vi "MGI RWA Unprocess Array Elements.vi"(0 "Queue In":refnum<queue>, 1 "Value":string, 2 "Read/Write Options":T2={"TS Fmt"="", "Int Fmt"="", "Delimiter"=","}, 3 "Format String (%#_13g)":string="%#_13g", 5 "Array Variant":variant, 7 "Name In":string, 9 "Str to INI in":variant, 11 "Error In":errorcluster, 12 "Use Specified?":bool, 13 "State In":T1={"StrToSpecifiedText"=variant, "Specified Data"=variant, "Float Fmt"="%#_13g", "Major Vers"=0, "Options"={"TS Fmt"="", "Int Fmt"="", "Delimiter"=","}}) -> (4 "Queue Out":refnum<queue>, 6 "Scan Failed?":bool, 8 "Data Out":string, 10 "Str to INI out":variant, 14 "State Out":T1={"StrToSpecifiedText"=variant, "Specified Data"=variant, "Float Fmt"="%#_13g", "Major Vers"=0, "Options"={"TS Fmt"="", "Int Fmt"="", "Delimiter"=","}}, 15 "Error Out":errorcluster)   [LabVIEW 2018]
doc: "This VI was created for use with the Read/Write Anything VIs. It finds any array elements that have been written to file and places their value in the array.\n\nAuthored by Robert C. Mortensen\nsupport@mooregoodideas.com\nwww.mooregoodideas.com\n\nCopyright (c) 2010, Moore Good Ideas, Inc.\n\nAll rights reserved.\n\nRedistribution and use in source and binary forms, with or without modification, are permitted provided that the following conditions are met:\n\n * Redistributions of source code must retain the above copyright notice, this list of conditions and the following disclaimer.\n * Redistributions in binary form must reproduce the above copyright notice, this list of conditions and the following disclaimer in the documentation and/or other materials provided with the distribution.\n * Neither the name of Moore Good Ideas, Inc. nor the names of its contributors may be used to endorse or promote products derived from this software without specific prior written permission.\n\nTHIS SOFTWARE IS PROVIDED BY THE COPYRIGHT HOLDERS AND CONTRIBUTORS \"AS IS\" AND ANY EXPRESS OR IMPLIED WARRANTIES, INCLUDING, BUT NOT LIMITED TO, THE IMPLIED WARRANTIES OF MERCHANTABILITY AND FITNESS FOR A PARTICULAR PURPOSE ARE DISCLAIMED. IN NO EVENT SHALL THE COPYRIGHT OWNER OR CONTRIBUTORS BE LIABLE FOR ANY DIRECT, INDIRECT, INCIDENTAL, SPECIAL, EXEMPLARY, OR CONSEQUENTIAL DAMAGES (INCLUDING, BUT NOT LIMITED TO, PROCUREMENT OF SUBSTITUTE GOODS OR SERVICES; LOSS OF USE, DATA, OR PROFITS; OR BUSINESS INTERRUPTION) HOWEVER CAUSED AND ON ANY THEORY OF LIABILITY, WHETHER IN CONTRACT, STRICT LIABILITY, OR TORT (INCLUDING NEGLIGENCE OR OTHERWISE) ARISING IN ANY WAY OUT OF THE USE OF THIS SOFTWARE, EVEN IF ADVISED OF THE POSSIBILITY OF SUCH DAMAGE."
uses:
  MGI RWA Tag Lookup Cluster.ctl
  MGI RWA Options Cluster.ctl
  MGI RWA Convertion Direction Enum.ctl
  MGI Scan From String (CSG[]).vi
  MGI Scan From String (CDB[]).vi
  MGI Scan From String (CXT[]).vi
  VariantType.lvlib
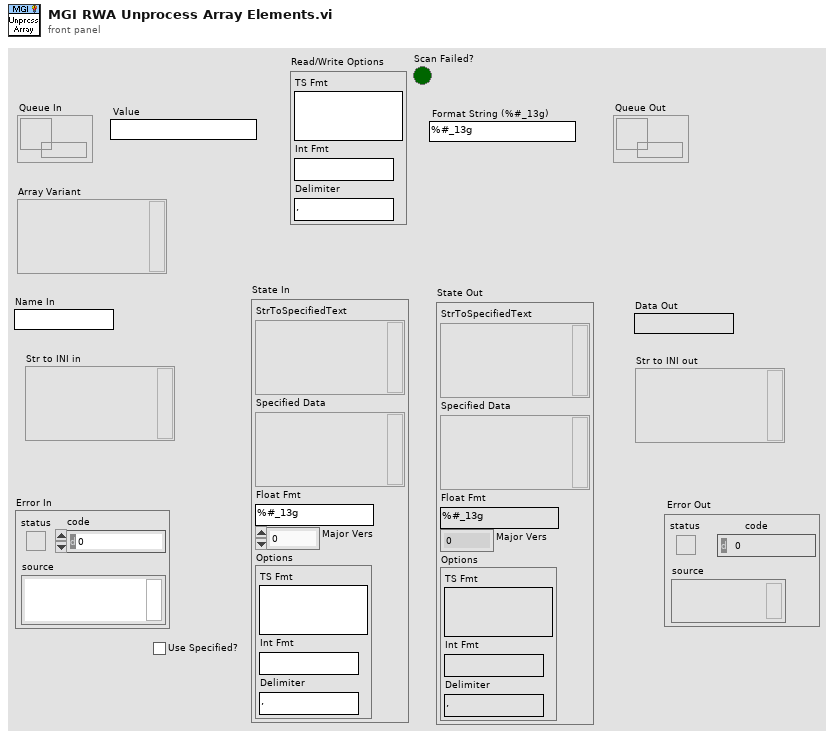
[diagram p1: front panel]
types:
  T1 = typedef "MGI RWA Tag Lookup Cluster.ctl" = cluster{"StrToSpecifiedText":variant, "Specified Data":variant, "Float Fmt":string, "Major Vers":i32, "Options":T2}
  T2 = typedef "MGI RWA Options Cluster.ctl" = cluster{"TS Fmt":string, "Int Fmt":string, "Delimiter":string}
  T3 = typedef "VariantType.lvlib/Type.ctl" = enum8{"Invalid Type", "Void", "I8", "I16", "I32", "I64", "U8", "U16", "U32", "U64", "Single Float", "Double Float", "Extended Float", "Single Complex", "Double Complex", "Extended Complex", "Enum U8", "Enum U16", "Enum U32", "Enum U64", "Single Float With Unit", "Double Float With Unit", "Extended Float With Unit", "Single Complex with Unit", "Double Complex with Unit", "Extended Complex with Unit", "Boolean", "String", "Path", "Picture", "Tag", "Array", "Cluster", "Variant", "LV Variant", "Waveform", "Timestamp", "Digital Waveform", "Digital Data", "ExpressData", "Refnum", "External Data", "VI", "Poly VI", "LabVIEW Class Instance", "Fixed Point"}
  T4 = typedef "MGI RWA Convertion Direction Enum.ctl" = enum16{"String->Anything", "Anything->String"}
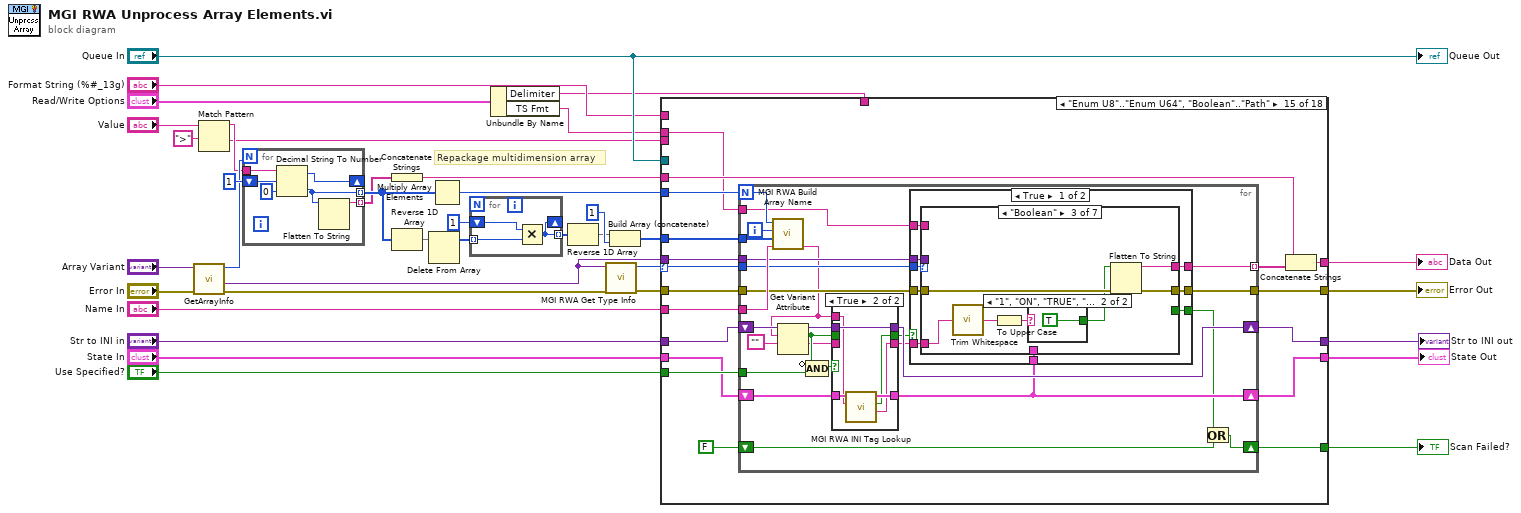
[diagram p0: block diagram]
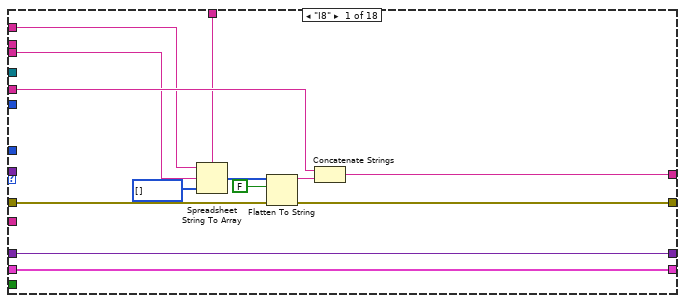
[diagram p2: hidden frame]
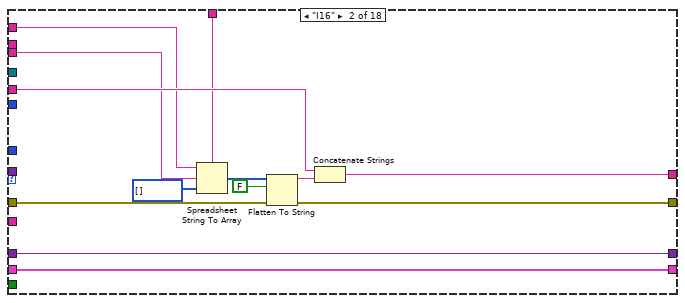
[diagram p3: hidden frame]
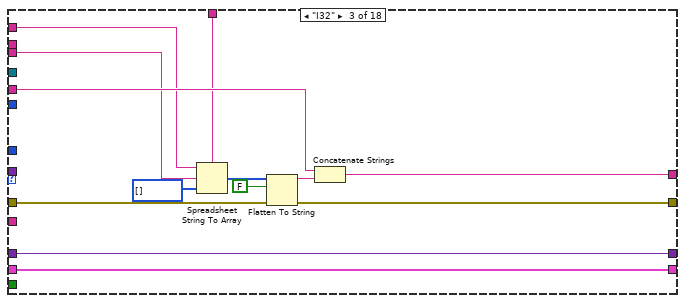
[diagram p4: hidden frame]
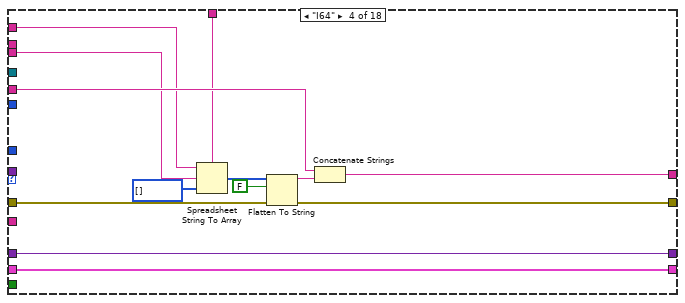
[diagram p5: hidden frame]
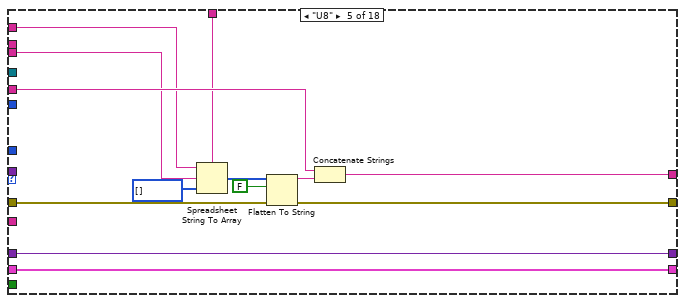
[diagram p6: hidden frame]
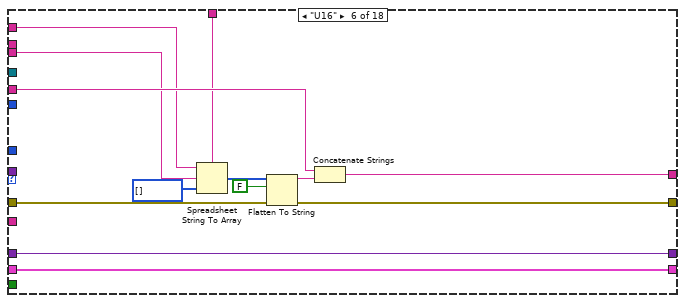
[diagram p7: hidden frame]
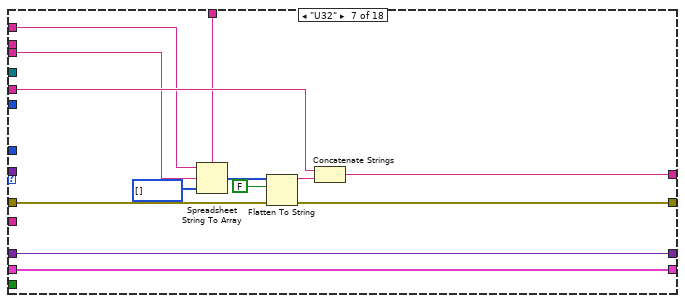
[diagram p8: hidden frame]
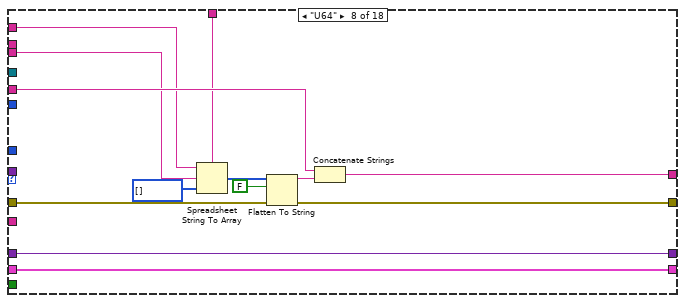
[diagram p9: hidden frame]
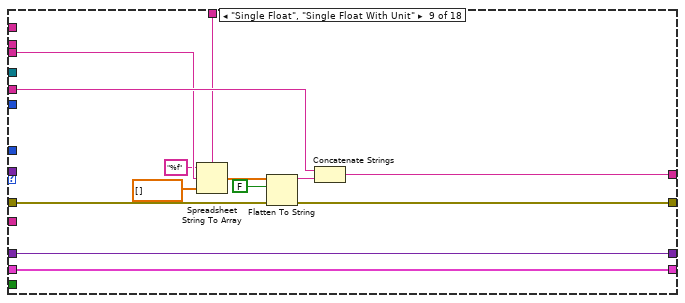
[diagram p10: hidden frame]
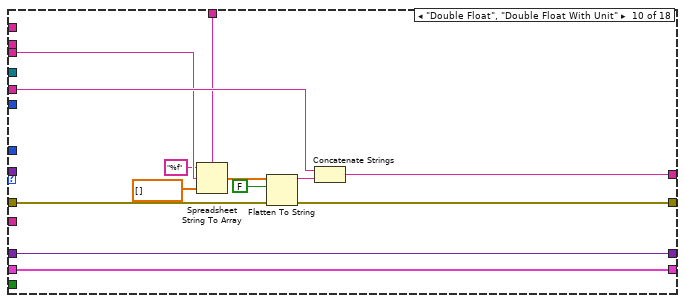
[diagram p11: hidden frame]
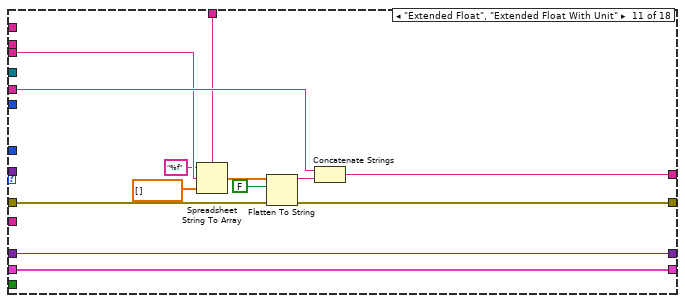
[diagram p12: hidden frame]
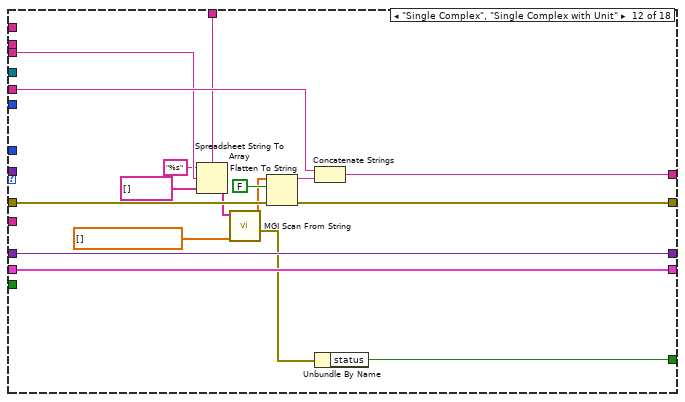
[diagram p13: hidden frame]
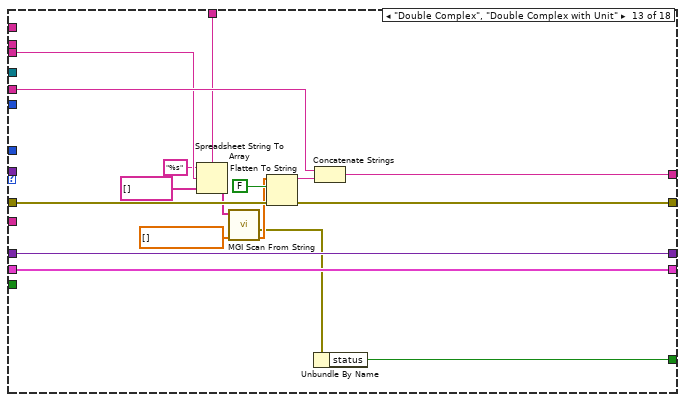
[diagram p14: hidden frame]
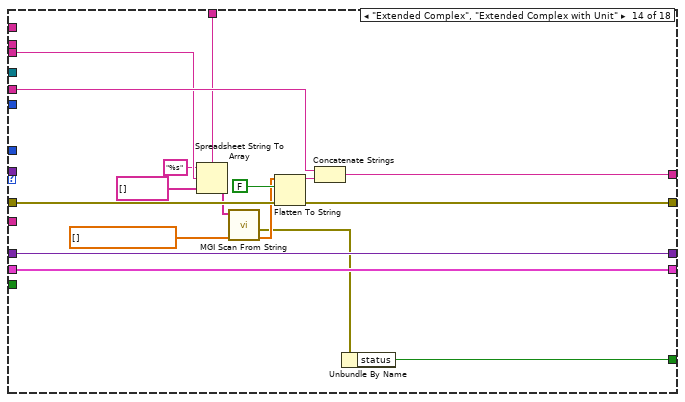
[diagram p15: hidden frame]
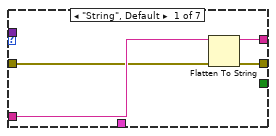
[diagram p17: hidden frame]
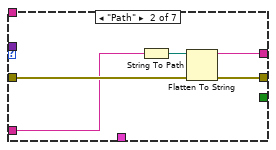
[diagram p18: hidden frame]
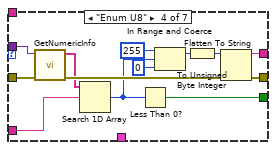
[diagram p20: hidden frame]
diagram:
  # "Repackage multidimension array"
  n1 = call "GetArrayInfo.vi"("error in (no error)"="Error In", "Variant"="Array Variant") -> ("error out"=w22:errorcluster, "ArrayElement"=w23:variant, "NDims"=w20:i32)  [unwired: 6 in, 1 out]
  n2 = Match Pattern(string="Value", regular expression=">") -> (before substring=w13:string, after substring=w12:string)  [unwired: 1 in, 2 out]
  n3 = for {
    N: w20 -> [_]
    shift-right: [w42] -> _
    shift-left: 1 ("offset past number") -> [w41]
    tunnel: w13 -> [w43]
    tunnel: [w39] -> w19 mode=indexing
    tunnel: [w38] -> w18 mode=indexing
    n4 = Decimal String To Number(string=w43, offset=w41, default (0L)=u32 0 ("default (0 I32)")) -> (offset past number=w42:i32, number=w39:u32)
    n5 = Flatten To String(anything=w39) -> (data string=w38:string)  [unwired: 3 in, 2 out]
  }
  n6 = Concatenate Strings(w18) -> (w17:string)
  n7 = Reverse 1D Array(array=w19) -> (reversed array=w27:u32[])
  n8 = Delete From Array(array=w27) -> (array with subset deleted=w28:u32[])  [unwired: 2 in, 1 out]
  n9 = Multiply Array Elements(1:w19) -> (0:w34:u32)
  n10 = for {
    tunnel: w28 -> [w46] mode=indexing
    shift-right: [w44] -> _
    shift-left: u32 1 -> [w45]
    tunnel: [w44] -> w30 mode=indexing
    n11 = Multiply(x=w45, y=w46) -> (x*y=w44:u32)
  }
  n12 = Unbundle By Name("Read/Write Options") -> ("Delimiter"=w3:string, "TS Fmt"=w4:string)
  n13 = Reverse 1D Array(array=w30) -> (reversed array=w31:u32[])
  n14 = call "MGI RWA Get Type Info.vi"("Error In"=w22, "Variant"=w23) -> ("Error Out"=w35:errorcluster, "Type Enum"=w2:T3)  [unwired: 7 in, 1 out]
  n15 = Build Array (concatenate)(w31, u32 1) -> (w26:u32[])
  n16 = case shown="\"Enum U8\"..\"Enum U64\", \"Boolean\"..\"Path\"" w2 {
    selector: w2 -> [_ _ _ _ _ _ _ _ _ _ _ _ _ _ w244 w414 _ _]
    tunnel: [w59 w72 w85 w98 w111 w124 w137 w150 w163 w176 w189 w206 w223 w240 w258 w426 w553 w590] -> w25
    tunnel: w35 -> [w58 w71 w84 w97 w110 w123 w136 w149 w162 w175 w188 w205 w222 w239 w257 w425 w560 w590]
    tunnel: w17 -> [w56 w69 w82 w95 w108 w121 w134 w147 w160 w173 w186 w203 w220 w237 w251 w420 w556 w588]
    tunnel: w34 -> [_ _ _ _ _ _ _ _ _ _ _ _ _ _ w256 w424 w559 _]
    tunnel: "Name In" -> [_ _ _ _ _ _ _ _ _ _ _ _ _ _ w255 w423 w558 _]
    tunnel: w26 -> [_ _ _ _ _ _ _ _ _ _ _ _ _ _ w254 w422 w557 _]
    tunnel: "Queue In" -> [_ _ _ _ _ _ _ _ _ _ _ _ _ _ _ _ w552 _]
    tunnel: w23 -> [_ _ _ _ _ _ _ _ _ _ _ _ _ _ w249 w418 w555 _]
    tunnel: "Str to INI in" -> [w48 w61 w74 w87 w100 w113 w126 w139 w152 w165 w178 w198 w214 w231 w253 w421 w549 w580]
    tunnel: [w57 w70 w83 w96 w109 w122 w135 w148 w161 w174 w187 w204 w221 w238 w250 w419 w556 w587] -> w16
    tunnel: w12 -> [w55 w68 w81 w94 w107 w120 w133 w146 w159 w172 w185 w202 w219 w236 _ w408 _ w578]
    tunnel: w3 -> [w50 w63 w76 w89 w102 w115 w128 w141 w153 w166 w179 w195 w215 w232 _ _ _ _]
    tunnel: "Format String (%#_13g)" -> [w49 w62 w75 w88 w101 w114 w127 w140 _ _ _ _ _ _ _ _ _ _]
    tunnel: [w48 w61 w74 w87 w100 w113 w126 w139 w152 w165 w178 w198 w214 w231 w248 w417 w549 w580] -> w7
    tunnel: "State In" -> [w47 w60 w73 w86 w99 w112 w125 w138 w151 w164 w177 w197 w213 w230 w246 w410 w548 w579]
    tunnel: "Use Specified?" -> [_ _ _ _ _ _ _ _ _ _ _ _ _ _ w247 w416 _ _]
    tunnel: [w47 w60 w73 w86 w99 w112 w125 w138 w151 w164 w177 w197 w213 w230 w245 w415 w548 w579] -> w8
    tunnel: w4 -> [_ _ _ _ _ _ _ _ _ _ _ _ _ _ w243 w413 _ _]
    tunnel: [_ _ _ _ _ _ _ _ _ _ _ w190 w207 w225 w241 w407 _ w575] -> w1
    frame "I8" {
      n17 = Spreadsheet String To Array(delimiter (Tab)=w50, format string=w49, spreadsheet string=w55, array type (2D Dbl)=i8[] []) -> (array=w54:i8[])
      n18 = Flatten To String(anything=w54, prepend array or string size? (T)=FALSE, error in (no error)=w58) -> (data string=w51:string, error out=w59:errorcluster)  [unwired: 1 in, 1 out]
      n19 = Concatenate Strings(w56, w51) -> (w57:string)
    }
    frame "I16" {
      n20 = Spreadsheet String To Array(delimiter (Tab)=w63, format string=w62, spreadsheet string=w68, array type (2D Dbl)=i16[] []) -> (array=w67:i16[])
      n21 = Flatten To String(anything=w67, prepend array or string size? (T)=FALSE, error in (no error)=w71) -> (data string=w64:string, error out=w72:errorcluster)  [unwired: 1 in, 1 out]
      n22 = Concatenate Strings(w69, w64) -> (w70:string)
    }
    frame "I32" {
      n23 = Spreadsheet String To Array(delimiter (Tab)=w76, format string=w75, spreadsheet string=w81, array type (2D Dbl)=i32[] []) -> (array=w80:i32[])
      n24 = Flatten To String(anything=w80, prepend array or string size? (T)=FALSE, error in (no error)=w84) -> (data string=w77:string, error out=w85:errorcluster)  [unwired: 1 in, 1 out]
      n25 = Concatenate Strings(w82, w77) -> (w83:string)
    }
    frame "I64" {
      n26 = Spreadsheet String To Array(delimiter (Tab)=w89, format string=w88, spreadsheet string=w94, array type (2D Dbl)=i64[] []) -> (array=w93:i64[])
      n27 = Flatten To String(anything=w93, prepend array or string size? (T)=FALSE, error in (no error)=w97) -> (data string=w90:string, error out=w98:errorcluster)  [unwired: 1 in, 1 out]
      n28 = Concatenate Strings(w95, w90) -> (w96:string)
    }
    frame "U8" {
      n29 = Spreadsheet String To Array(delimiter (Tab)=w102, format string=w101, spreadsheet string=w107, array type (2D Dbl)=u8[] []) -> (array=w106:u8[])
      n30 = Flatten To String(anything=w106, prepend array or string size? (T)=FALSE, error in (no error)=w110) -> (data string=w103:string, error out=w111:errorcluster)  [unwired: 1 in, 1 out]
      n31 = Concatenate Strings(w108, w103) -> (w109:string)
    }
    frame "U16" {
      n32 = Spreadsheet String To Array(delimiter (Tab)=w115, format string=w114, spreadsheet string=w120, array type (2D Dbl)=u16[] []) -> (array=w119:u16[])
      n33 = Flatten To String(anything=w119, prepend array or string size? (T)=FALSE, error in (no error)=w123) -> (data string=w116:string, error out=w124:errorcluster)  [unwired: 1 in, 1 out]
      n34 = Concatenate Strings(w121, w116) -> (w122:string)
    }
    frame "U32" {
      n35 = Spreadsheet String To Array(delimiter (Tab)=w128, format string=w127, spreadsheet string=w133, array type (2D Dbl)=u32[] []) -> (array=w132:u32[])
      n36 = Flatten To String(anything=w132, prepend array or string size? (T)=FALSE, error in (no error)=w136) -> (data string=w129:string, error out=w137:errorcluster)  [unwired: 1 in, 1 out]
      n37 = Concatenate Strings(w134, w129) -> (w135:string)
    }
    frame "U64" {
      n38 = Spreadsheet String To Array(delimiter (Tab)=w141, format string=w140, spreadsheet string=w146, array type (2D Dbl)=u64[] []) -> (array=w145:u64[])
      n39 = Flatten To String(anything=w145, prepend array or string size? (T)=FALSE, error in (no error)=w149) -> (data string=w142:string, error out=w150:errorcluster)  [unwired: 1 in, 1 out]
      n40 = Concatenate Strings(w147, w142) -> (w148:string)
    }
    frame "Single Float", "Single Float With Unit" {
      n41 = Spreadsheet String To Array(delimiter (Tab)=w153, format string="%f", spreadsheet string=w159, array type (2D Dbl)=sgl[] []) -> (array=w157:sgl[])
      n42 = Flatten To String(anything=w157, prepend array or string size? (T)=FALSE, error in (no error)=w162) -> (data string=w154:string, error out=w163:errorcluster)  [unwired: 1 in, 1 out]
      n43 = Concatenate Strings(w160, w154) -> (w161:string)
    }
    frame "Double Float", "Double Float With Unit" {
      n44 = Spreadsheet String To Array(delimiter (Tab)=w166, format string="%f", spreadsheet string=w172, array type (2D Dbl)=dbl[] []) -> (array=w170:dbl[])
      n45 = Flatten To String(anything=w170, prepend array or string size? (T)=FALSE, error in (no error)=w175) -> (data string=w167:string, error out=w176:errorcluster)  [unwired: 1 in, 1 out]
      n46 = Concatenate Strings(w173, w167) -> (w174:string)
    }
    frame "Extended Float", "Extended Float With Unit" {
      n47 = Spreadsheet String To Array(delimiter (Tab)=w179, format string="%f", spreadsheet string=w185, array type (2D Dbl)=ext[] []) -> (array=w183:ext[])
      n48 = Flatten To String(anything=w183, prepend array or string size? (T)=FALSE, error in (no error)=w188) -> (data string=w180:string, error out=w189:errorcluster)  [unwired: 1 in, 1 out]
      n49 = Concatenate Strings(w186, w180) -> (w187:string)
    }
    frame "Single Complex", "Single Complex with Unit" {
      n50 = Spreadsheet String To Array(delimiter (Tab)=w195, format string="%s", spreadsheet string=w202, array type (2D Dbl)=string[] [] ("String[]")) -> (array=w193:string[])
      n51 = call-poly "MGI Scan From String.vi"("Default CSG[]"=csg[] [], "String[]"=w193) -> ("CSG[] Out"=w192:csg[], "error out"=w191:errorcluster)  [unwired: 8 in]
      n52 = Flatten To String(anything=w192, prepend array or string size? (T)=FALSE, error in (no error)=w205) -> (data string=w199:string, error out=w206:errorcluster)  [unwired: 1 in, 1 out]
      n53 = Concatenate Strings(w203, w199) -> (w204:string)
      n54 = Unbundle By Name(w191) -> ("status"=w190:bool)
    }
    frame "Double Complex", "Double Complex with Unit" {
      n55 = Spreadsheet String To Array(delimiter (Tab)=w215, format string="%s", spreadsheet string=w219, array type (2D Dbl)=string[] [] ("String[]")) -> (array=w212:string[])
      n56 = call-poly "MGI Scan From String.vi"("Default CDB[]"=cdb[] [] ("Default DBL[]"), "String[]"=w212) -> ("CDB[] Out"=w209:cdb[], "error out"=w208:errorcluster)  [unwired: 8 in]
      n57 = Flatten To String(anything=w209, prepend array or string size? (T)=FALSE, error in (no error)=w222) -> (data string=w216:string, error out=w223:errorcluster)  [unwired: 1 in, 1 out]
      n58 = Unbundle By Name(w208) -> ("status"=w207:bool)
      n59 = Concatenate Strings(w220, w216) -> (w221:string)
    }
    frame "Extended Complex", "Extended Complex with Unit" {
      n60 = Spreadsheet String To Array(delimiter (Tab)=w232, format string="%s", spreadsheet string=w236, array type (2D Dbl)=string[] [] ("String[]")) -> (array=w228:string[])
      n61 = call-poly "MGI Scan From String.vi"("Default CXT[]"=cxt[] [] ("Default DBL[]"), "String[]"=w228) -> ("CXT[] Out"=w227:cxt[], "error out"=w226:errorcluster)  [unwired: 8 in]
      n62 = Flatten To String(anything=w227, prepend array or string size? (T)=FALSE, error in (no error)=w239) -> (data string=w233:string, error out=w240:errorcluster)  [unwired: 1 in, 1 out]
      n63 = Concatenate Strings(w237, w233) -> (w238:string)
      n64 = Unbundle By Name(w226) -> ("status"=w225:bool)
    }
    frame "Enum U8".."Enum U64", "Boolean".."Path" {
      n65 = for {
        N: w256 -> [w284]
        tunnel: [w279] -> w258
        tunnel: w257 -> [w280]
        tunnel: w255 -> [w281]
        tunnel: w254 -> [w282]
        tunnel: [w278] -> w252 mode=indexing
        tunnel: w249 -> [w277]
        shift-right: [w268] -> w248
        shift-left: w253 -> [w272]
        tunnel: w247 -> [w271]
        shift-right: [w262] -> w245
        shift-left: w246 -> [w269]
        tunnel: w244 -> [w265]
        tunnel: w243 -> [w263]
        shift-right: [w259] -> w241
        shift-left: FALSE -> [w261]
        i -> [w283]
        n66 = call "MGI RWA Build Array Name.vi"("Name In"=w281, "Array"=w282, "Iteration"=w283, "Iterations"=w284) -> ("Name Out"=w264:string)  [unwired: 7 in]
        n67 = Get Variant Attribute(Variant=w272, name=w264, default value (empty Variant)="") -> (duplicate Variant=w276:variant, found=w275:bool, value=w274:string)  [unwired: 1 in, 1 out]
        n68 = Compound Arithmetic op=AND(invert w275, w271) -> (w270:bool)
        n69 = case shown="True" w270 {
          tunnel: w274 -> [w286 _]
          tunnel: w275 -> [w287 _]
          tunnel: w264 -> [_ w289]
          tunnel: w276 -> [w288 w293]
          tunnel: [w288 w293] -> w268
          tunnel: [w287 w291] -> w267
          tunnel: [w286 w290] -> w266
          tunnel: w269 -> [w285 w294]
          tunnel: [w285 w292] -> w262
          frame False {
          }
          frame True {
            n70 = call "MGI RWA INI Tag Lookup.vi"("String"=w289, "State In"=w294) -> ("INI Text"=w290:string, "Text Found?"=w291:bool, "State Out"=w292:T1)  [unwired: 7 in]
          }
        }
        n71 = case shown="True" w267 {
          tunnel: [w302 w376] -> w279
          tunnel: w280 -> [w301 w377]
          tunnel: [w303 w378] -> w278
          tunnel: w277 -> [w300 w373]
          tunnel: w266 -> [w299 _]
          tunnel: w265 -> [w298 w375]
          tunnel: w263 -> [w297 _]
          tunnel: w262 -> [w296 w374]
          tunnel: [w295 _] -> w260
          frame True {
            n72 = case shown="\"Boolean\"" w298 {
              tunnel: [w304 w309 w318 w333 w346 w359 w372] -> w303
              tunnel: [w305 w310 w317 w332 w345 w358 w371] -> w302
              tunnel: w301 -> [w306 w311 w319 w331 w344 w357 w370]
              tunnel: w300 -> [_ _ _ w330 w343 w356 w369]
              tunnel: w299 -> [w307 w308 w314 w327 w340 w353 w366]
              tunnel: w297 -> [_ _ _ _ _ _ _]
              tunnel: w296 -> [_ _ _ _ _ _ _]
              tunnel: [_ _ _ w321 w334 w347 w360] -> w295
              frame "String", Default {
                n73 = Flatten To String(anything=w307, error in (no error)=w306) -> (data string=w304:string, error out=w305:errorcluster)  [unwired: 2 in, 1 out]
              }
              frame "Path" {
                n74 = String To Path(string=w308) -> (path=w312:path)
                n75 = Flatten To String(anything=w312, error in (no error)=w311) -> (data string=w309:string, error out=w310:errorcluster)  [unwired: 2 in, 1 out]
              }
              frame "Boolean" {
                n76 = call "Trim Whitespace.vi"("string"=w314) -> ("trimmed string"=w315:string)  [unwired: 1 in]
                n77 = To Upper Case(1:w315) -> (0:w316:string)
                n78 = case shown="\"1\", \"ON\", \"TRUE\", \"YES\"" w316 {
                  tunnel: [_ TRUE] -> w313
                  frame Default {
                  }
                  frame "1", "ON", "TRUE", "YES" {
                  }
                }
                n79 = Flatten To String(anything=w313, error in (no error)=w319) -> (data string=w318:string, error out=w317:errorcluster)  [unwired: 2 in, 1 out]
              }
              frame "Enum U8" {
                n80 = call "GetNumericInfo.vi"("error in (no error)"=w331, "Variant"=w330) -> ("error out"=w329:errorcluster, "EnumNames"=w328:string[])  [unwired: 6 in, 2 out]
                n81 = Search 1D Array(1D array=w328, element=w327) -> (index of element=w322:i32)  [unwired: 1 in]
                n82 = Less Than 0?(x=w322) -> (x < 0?=w321:bool)
                n83 = In Range and Coerce(upper limit=255, x=w322, lower limit=0) -> (coerced(x)=w326:i32)  [unwired: 1 out]
                n84 = To Unsigned Byte Integer(number=w326) -> (unsigned 8bit integer=w325:u8)
                n85 = Flatten To String(anything=w325, error in (no error)=w329) -> (data string=w333:string, error out=w332:errorcluster)  [unwired: 2 in, 1 out]
              }
              frame "Enum U16" {
                n86 = call "GetNumericInfo.vi"("error in (no error)"=w344, "Variant"=w343) -> ("error out"=w342:errorcluster, "EnumNames"=w341:string[])  [unwired: 6 in, 2 out]
                n87 = Search 1D Array(1D array=w341, element=w340) -> (index of element=w335:i32)  [unwired: 1 in]
                n88 = Less Than 0?(x=w335) -> (x < 0?=w334:bool)
                n89 = In Range and Coerce(upper limit=65535, x=w335, lower limit=0) -> (coerced(x)=w339:i32)  [unwired: 1 out]
                n90 = To Unsigned Word Integer(number=w339) -> (unsigned 16bit integer=w338:u16)
                n91 = Flatten To String(anything=w338, error in (no error)=w342) -> (data string=w346:string, error out=w345:errorcluster)  [unwired: 2 in, 1 out]
              }
              frame "Enum U32" {
                n92 = call "GetNumericInfo.vi"("error in (no error)"=w357, "Variant"=w356) -> ("error out"=w355:errorcluster, "EnumNames"=w354:string[])  [unwired: 6 in, 2 out]
                n93 = Search 1D Array(1D array=w354, element=w353) -> (index of element=w348:i32)  [unwired: 1 in]
                n94 = Less Than 0?(x=w348) -> (x < 0?=w347:bool)
                n95 = In Range and Coerce(upper limit=2147483647, x=w348, lower limit=0) -> (coerced(x)=w352:i32)  [unwired: 1 out]
                n96 = To Unsigned Long Integer(number=w352) -> (unsigned 32bit integer=w351:u32)
                n97 = Flatten To String(anything=w351, error in (no error)=w355) -> (data string=w359:string, error out=w358:errorcluster)  [unwired: 2 in, 1 out]
              }
              frame "Enum U64" {
                n98 = call "GetNumericInfo.vi"("error in (no error)"=w370, "Variant"=w369) -> ("error out"=w368:errorcluster, "EnumNames"=w367:string[])  [unwired: 6 in, 2 out]
                n99 = Search 1D Array(1D array=w367, element=w366) -> (index of element=w361:i32)  [unwired: 1 in]
                n100 = Less Than 0?(x=w361) -> (x < 0?=w360:bool)
                n101 = In Range and Coerce(upper limit=2147483647, x=w361, lower limit=0) -> (coerced(x)=w364:i32)  [unwired: 1 out]
                n102 = To Unsigned Quad Integer(1:w364) -> (0:w363:u64)
                n103 = Flatten To String(anything=w363, error in (no error)=w368) -> (data string=w372:string, error out=w371:errorcluster)  [unwired: 2 in, 1 out]
              }
            }
          }
          frame False {
            n104 = case shown="\"Path\"" w375 {
              tunnel: [w379 w385 w387 w394 w398 w402 w406] -> w378
              tunnel: w377 -> [w381 w383 w389 w392 w396 w400 w404]
              tunnel: [w380 w384 w388 w391 w395 w399 w403] -> w376
              tunnel: w374 -> [_ _ _ _ _ _ _]
              tunnel: w373 -> [_ _ _ _ _ _ _]
              frame "String", Default {
                n105 = Flatten To String(anything="", error in (no error)=w381) -> (data string=w379:string, error out=w380:errorcluster)  [unwired: 2 in, 1 out]
              }
              frame "Path" {
                n106 = Flatten To String(anything=path "", error in (no error)=w383) -> (data string=w385:string, error out=w384:errorcluster)  [unwired: 2 in, 1 out]
              }
              frame "Boolean" {
                n107 = Flatten To String(anything=FALSE, error in (no error)=w389) -> (data string=w387:string, error out=w388:errorcluster)  [unwired: 2 in, 1 out]
              }
              frame "Enum U8" {
                n108 = Flatten To String(anything=u8 0, error in (no error)=w392) -> (data string=w394:string, error out=w391:errorcluster)  [unwired: 2 in, 1 out]
              }
              frame "Enum U16" {
                n109 = Flatten To String(anything=u16 0, error in (no error)=w396) -> (data string=w398:string, error out=w395:errorcluster)  [unwired: 2 in, 1 out]
              }
              frame "Enum U32" {
                n110 = Flatten To String(anything=u32 0, error in (no error)=w400) -> (data string=w402:string, error out=w399:errorcluster)  [unwired: 2 in, 1 out]
              }
              frame "Enum U64" {
                n111 = Flatten To String(anything=u64 0, error in (no error)=w404) -> (data string=w406:string, error out=w403:errorcluster)  [unwired: 2 in, 1 out]
              }
            }
          }
        }
        n112 = Or(x=w260, y=w261) -> (x .or. y?=w259:bool)
      }
      n113 = Concatenate Strings(w251, w252) -> (w250:string)
    }
    frame "Tag", "Timestamp", "Refnum" {
      # "Version 1.0 writes Tag,Timestamp, and Refnum as a hex string"
      n114 = Unbundle By Name(w410) -> ("Major Vers"=w412:i32)
      n115 = Less?(x=w412, y=2) -> (x < y?=w409:bool)
      n116 = case shown="False" w409 {
        tunnel: [w444 w541] -> w426
        tunnel: w425 -> [w443 w541]
        tunnel: w424 -> [w442 _]
        tunnel: w423 -> [w441 _]
        tunnel: w422 -> [w440 _]
        tunnel: w421 -> [w439 w542]
        tunnel: w420 -> [w437 w544]
        tunnel: [w436 w543] -> w419
        tunnel: w418 -> [w435 _]
        tunnel: [w434 w542] -> w417
        tunnel: w416 -> [w433 _]
        tunnel: [w432 w545] -> w415
        tunnel: w414 -> [w431 _]
        tunnel: w413 -> [w430 _]
        tunnel: w410 -> [w429 w545]
        tunnel: w408 -> [_ w538]
        tunnel: [w427 _] -> w407
        frame False {
          n117 = for {
            N: w442 -> [w470]
            tunnel: [w465] -> w444
            tunnel: w443 -> [w466]
            tunnel: w441 -> [w467]
            tunnel: w440 -> [w468]
            tunnel: [w464] -> w438 mode=indexing
            tunnel: w435 -> [w463]
            shift-right: [w454] -> w434
            shift-left: w439 -> [w458]
            tunnel: w433 -> [w457]
            shift-right: [w448] -> w432
            shift-left: w429 -> [w455]
            tunnel: w431 -> [w451]
            tunnel: w430 -> [w449]
            shift-right: [w446] -> w427
            shift-left: FALSE -> [w447]
            i -> [w469]
            n118 = call "MGI RWA Build Array Name.vi"("Name In"=w467, "Array"=w468, "Iteration"=w469, "Iterations"=w470) -> ("Name Out"=w450:string)  [unwired: 7 in]
            n119 = Get Variant Attribute(Variant=w458, name=w450, default value (empty Variant)="") -> (duplicate Variant=w462:variant, found=w461:bool, value=w460:string)  [unwired: 1 in, 1 out]
            n120 = Compound Arithmetic op=AND(invert w461, w457) -> (w456:bool)
            n121 = case shown="True" w456 {
              tunnel: w460 -> [w472 _]
              tunnel: w461 -> [w473 _]
              tunnel: w450 -> [_ w475]
              tunnel: w462 -> [w474 w479]
              tunnel: [w474 w479] -> w454
              tunnel: [w473 w477] -> w453
              tunnel: [w472 w476] -> w452
              tunnel: w455 -> [w471 w480]
              tunnel: [w471 w478] -> w448
              frame False {
              }
              frame True {
                n122 = call "MGI RWA INI Tag Lookup.vi"("String"=w475, "State In"=w480) -> ("INI Text"=w476:string, "Text Found?"=w477:bool, "State Out"=w478:T1)  [unwired: 7 in]
              }
            }
            n123 = case shown="False" w453 {
              tunnel: [w488 w525] -> w465
              tunnel: w466 -> [w487 w526]
              tunnel: [w489 w527] -> w464
              tunnel: w463 -> [w486 w522]
              tunnel: w452 -> [w485 _]
              tunnel: w451 -> [w484 w524]
              tunnel: w449 -> [w483 _]
              tunnel: w448 -> [w482 w523]
              tunnel: [w481 _] -> w445
              frame True {
                n124 = case shown="\"Timestamp\", Default" w484 {
                  tunnel: [w494 w518] -> w489
                  tunnel: [w495 w516] -> w488
                  tunnel: w487 -> [w492 w516]
                  tunnel: w486 -> [_ w521]
                  tunnel: w485 -> [w493 w519]
                  tunnel: w483 -> [w491 _]
                  tunnel: w482 -> [_ w520]
                  tunnel: [w490 w514] -> w481
                  frame "Timestamp", Default {
                    n125 = case shown="Default" w491 {
                      selector: w491 -> [_ w505]
                      tunnel: [w498 w513] -> w495
                      tunnel: [w496 w512] -> w494
                      tunnel: w493 -> [w497 w511]
                      tunnel: w492 -> [w498 w504]
                      tunnel: [_ w502] -> w490
                      frame "" {
                        n126 = String Subset(string=w497, offset (0)=2) -> (substring=w500:string)  [unwired: 1 in]
                        n127 = call "MGI Hex Str to U8 Data.vi"("HEX String (0-9,A-F)"=w500) -> ("u8 Data[]"=w499:u8[])
                        n128 = Byte Array To String(unsigned byte array=w499) -> (string=w496:string)
                      }
                      frame Default {
                        n129 = Concatenate Strings("%<" ("string"), w505, ">T" ("string")) -> (w508:string)
                        n130 = Scan From String(format string=w508, input string=w511, default 1=timestamp(0 s since 1904-01-01)) -> (error out=w503:errorcluster, output 1=w510:timestamp)  [unwired: 2 in, 2 out]
                        n131 = Unbundle(w503) -> ("status"=w502:bool)  [unwired: 2 out]
                        n132 = Flatten To String(anything=w510, error in (no error)=w504) -> (data string=w512:string, error out=w513:errorcluster)  [unwired: 2 in, 1 out]
                      }
                    }
                  }
                  frame "Tag", "Refnum" {
                    n133 = call "MGI RWA Handle Tag or Refnum.vi"("Read State In"=w520, "Conversion"=MGI_RWA_Convertion_Direction_Enum."String->Anything", "Anything"=w521, "Read String"=w519) -> ("Error Out"=w515:errorcluster, "String"=w518:string)  [unwired: 6 in]
                    n134 = Unbundle By Name(w515) -> ("status"=w514:bool)
                  }
                }
              }
              frame False {
                n135 = case shown="\"Tag\", \"Refnum\"" w524 {
                  tunnel: [w531 w536] -> w527
                  tunnel: w526 -> [w529 w532]
                  tunnel: [w530 w532] -> w525
                  tunnel: w523 -> [_ w537]
                  tunnel: w522 -> [_ w534]
                  frame "Timestamp", Default {
                    n136 = Flatten To String(anything=timestamp(0 s since 1904-01-01), error in (no error)=w529) -> (data string=w531:string, error out=w530:errorcluster)  [unwired: 2 in, 1 out]
                  }
                  frame "Tag", "Refnum" {
                    n137 = call "MGI RWA Handle Tag or Refnum.vi"("Read State In"=w537, "Conversion"=MGI_RWA_Convertion_Direction_Enum."String->Anything", "Error In"=w532, "Anything"=w534, "Read String"="") -> ("String"=w536:string)  [unwired: 5 in, 1 out]
                  }
                }
              }
            }
            n138 = Or(x=w445, y=w447) -> (x .or. y?=w446:bool)
          }
          n139 = Concatenate Strings(w437, w438) -> (w436:string)
        }
        frame True {
          n140 = String Subset(string=w538, offset (0)=2) -> (substring=w540:string)  [unwired: 1 in]
          n141 = call "MGI Hex Str to U8 Data.vi"("HEX String (0-9,A-F)"=w540) -> ("u8 Data[]"=w539:u8[])
          n142 = Byte Array To String(unsigned byte array=w539) -> (string=w547:string)
          n143 = Concatenate Strings(w544, w547) -> (w543:string)
        }
      }
    }
    frame "Cluster" {
      # "Enqueue cluster element"
      n144 = for {
        N: w559 -> [w574]
        tunnel: w560 -> [w566]
        tunnel: w558 -> [w571]
        tunnel: w557 -> [w572]
        tunnel: w555 -> [w567]
        tunnel: [w566] -> w554
        tunnel: [w565] -> w551 mode=indexing
        i -> [w573]
        n145 = call "MGI RWA Build Array Name.vi"("Name In"=w571, "Array"=w572, "Iteration"=w573, "Iterations"=w574) -> ("Name Out"=w568:string)  [unwired: 7 in]
        n146 = Concatenate Strings(w568, "." ("string")) -> (w570:string)
        n147 = Bundle("ArrayElement"=w567, w570) -> (w565:cluster{"ArrayElement":variant, string})  [unwired: 1 in]
      }
      n148 = Reverse 1D Array(array=w551) -> (reversed array=w550:cluster{"ArrayElement":variant, string}[])
      n149 = for {
        tunnel: w554 -> [w564]
        tunnel: [w563] -> w553
        tunnel: w552 -> [w562]
        tunnel: w550 -> [w561] mode=indexing
        n150 = Enqueue Element At Opposite End(queue=w562, element=w561, error in (no error)=w564) -> (error out=w563:errorcluster)  [unwired: 1 in, 2 out]
      }
    }
    frame Default {
      n151 = String Subset(string=w578, offset (0)=2) -> (substring=w584:string)  [unwired: 1 in]
      n152 = Search/Split String(string=w578, search string/char (-)="0x") -> (offset of match=w576:i32)  [unwired: 1 in, 2 out]
      n153 = String Length(string=w584) -> (length=w585:i32)
      n154 = Less Than 0?(x=w576) -> (x < 0?=w575:bool)
      n155 = Multiply(x=0.5, y=w585) -> (x*y=w586:dbl)
      n156 = for {
        N: w586 -> [_]
        tunnel: w584 -> [w594]
        tunnel: [w596] -> w582 mode=indexing
        i -> [w593]
        w592 = 2 ("length (rest)")
        n157 = Multiply(x=w593, y=w592) -> (x*y=w591:i32)
        n158 = String Subset(string=w594, offset (0)=w591, length (rest)=w592) -> (substring=w595:string)
        n159 = Hexadecimal String To Number(string=w595, default (0uL)=u8 0 ("default (0 U32)")) -> (number=w596:u8)  [unwired: 1 in, 1 out]
      }
      n160 = Byte Array To String(unsigned byte array=w582) -> (string=w589:string)
      n161 = Concatenate Strings(w588, w589) -> (w587:string)
    }
  }
  "Error Out" <- w25
  "Data Out" <- w16
  "State Out" <- w8
  "Str to INI out" <- w7
  "Scan Failed?" <- w1
  "Queue Out" <- "Queue In"
